vi "Диалог_на_Макро.vi"(8 "АДРЕС ДЛЯ ЗАПИСИ ДА":string, 9 "АДРЕС ДЛЯ ЗАПИСИ НЕТ":string, 11 "ОПИСАНИЕ":string) -> ()   [LabVIEW 2011]
panel:
  in  "НЕТ":bool
  in  "ДА":bool
  out "ВОПРОС":string
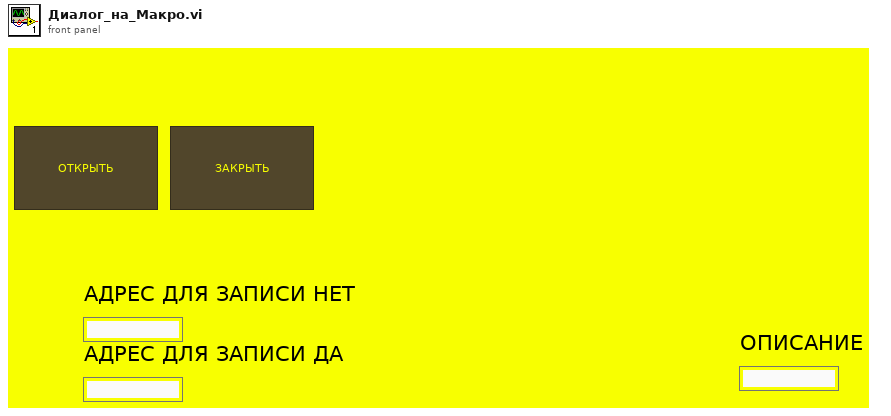
[diagram p1: front panel]
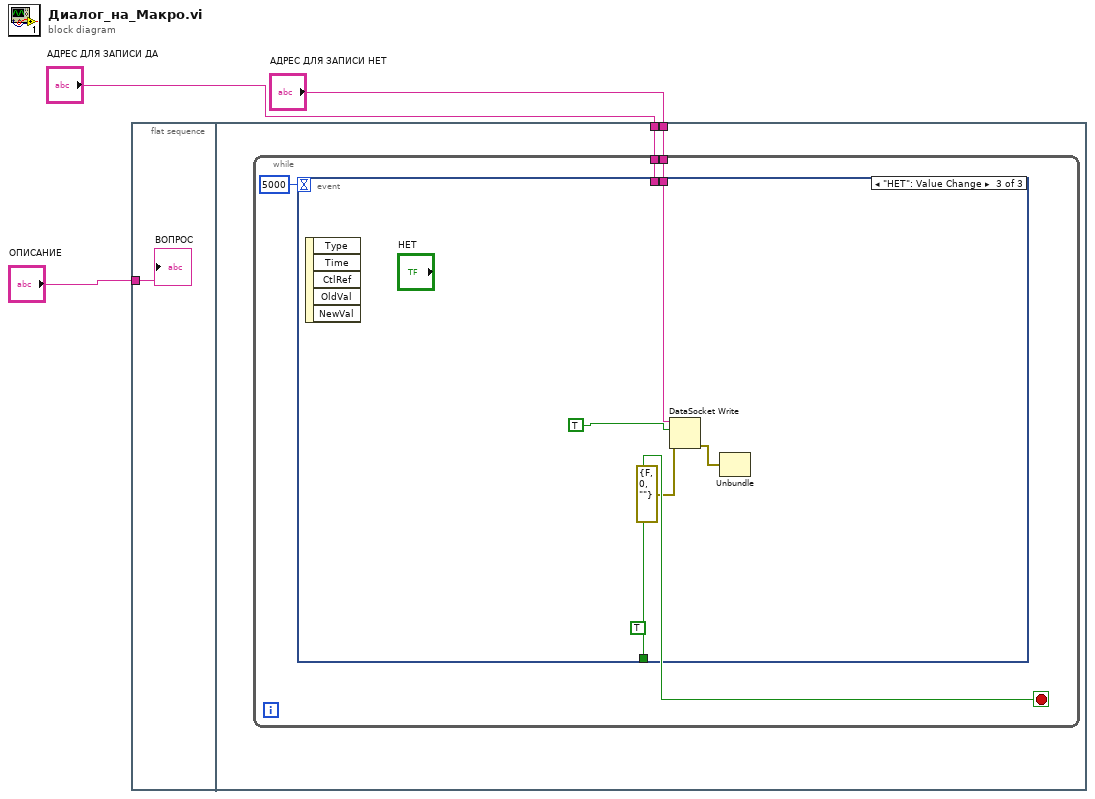
[diagram p0: block diagram]
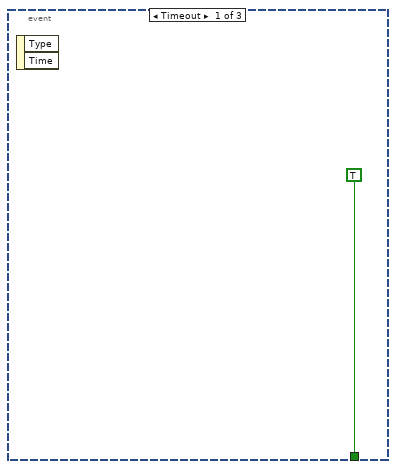
[diagram p2: hidden frame]
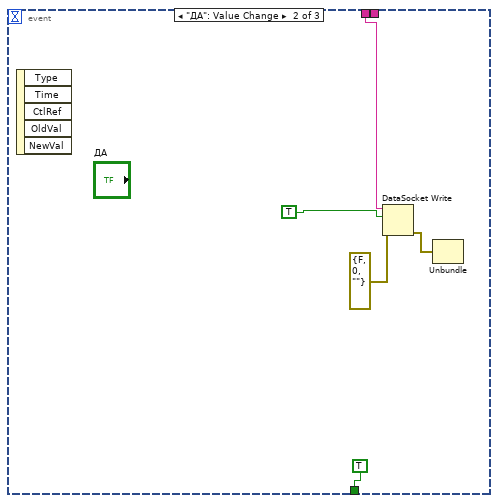
[diagram p3: hidden frame]
diagram:
  n1 = flat-sequence {
    tunnel: "ОПИСАНИЕ" -> [w4]
    tunnel: "АДРЕС ДЛЯ ЗАПИСИ НЕТ" -> [w6]
    tunnel: "АДРЕС ДЛЯ ЗАПИСИ ДА" -> [w5]
    frame #0 {
      "ВОПРОС" <- w4
    }
    frame #1 {
      n2 = while {
        tunnel: w6 -> [w8]
        tunnel: w5 -> [w7]
        stop <- w10 stop-if-true
        n3 = event shown="[2] \"НЕТ\": Value Change" {
          selector: _ -> [_ _ _]
          dyn-events: _ -> [_ _ _]
          timeout: 5000 -> [_ _ _]
          tunnel: [TRUE ("Boolean") TRUE ("Boolean") TRUE ("Boolean")] -> w10
          tunnel: w8 -> [_ _ w17]
          tunnel: w7 -> [_ w12 _]
          event Timeout {
            n4 = event-data() -> ()  [unwired: 1 in, 2 out]
          }
          event "ДА": Value Change {
            n5 = event-data() -> ()  [unwired: 1 in, 5 out]
            n6 = DataSocket Write(8:errorcluster {"status"=FALSE, "code"=0, "source"=""} ("error in (no error)"), 10:TRUE, 11:w12) -> (0:w14:errorcluster)  [unwired: 1 in, 2 out]
            n7 = Unbundle(w14) -> ()  [unwired: 3 out]
          }
          event "НЕТ": Value Change {
            n8 = event-data() -> ()  [unwired: 1 in, 5 out]
            n9 = DataSocket Write(8:errorcluster {"status"=FALSE, "code"=0, "source"=""} ("error in (no error)"), 10:TRUE, 11:w17) -> (0:w19:errorcluster)  [unwired: 1 in, 2 out]
            n10 = Unbundle(w19) -> ()  [unwired: 3 out]
          }
        }
      }
    }
  }
